vi "Set PPMS parameter.vi"(8 "error in (no error)":errorcluster, 9 "Input Value":variant, 10 "Control Name":string, 11 "VI reference in":refnum<vi>) -> (0 "error out":errorcluster, 3 "VI reference out":refnum<vi>)   [LabVIEW 2025]
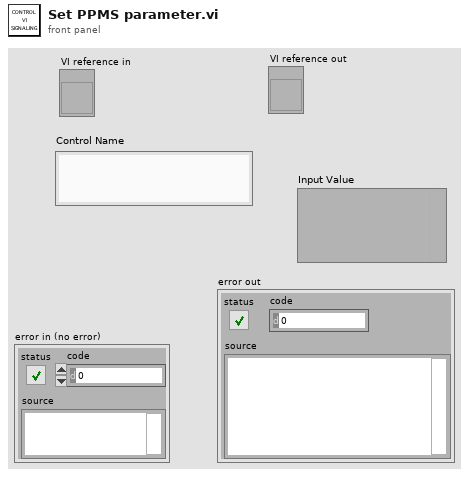
[diagram p1: front panel]
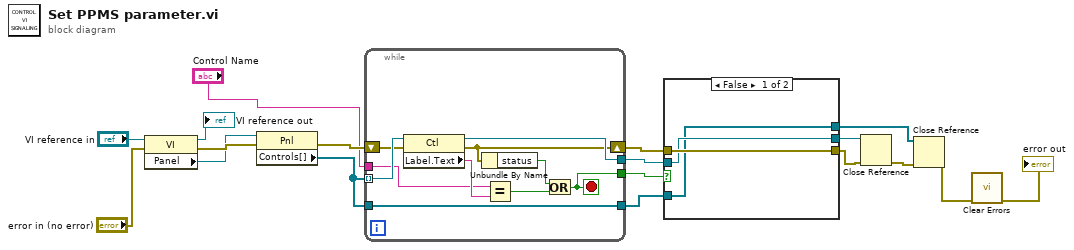
[diagram p0: block diagram]
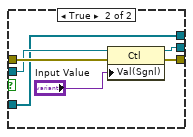
[diagram p2: hidden frame]
diagram:
  n1 = property class="VI"(reference="VI reference in", error in="error in (no error)") -> (reference out=→"VI reference out":refnum<vi>, error out=w18:errorcluster, "Panel"=w11:refnum<vi>)
  n2 = property class="Pnl"(reference=w11, error in=w18) -> (error out=w17:errorcluster, "Controls[]"=w13:refnum<vi>[])  [unwired: 1 out]
  n3 = while {
    tunnel: w13 -> [w28] mode=indexing
    tunnel: "Control Name" -> [w26]
    shift-right: [w23] -> w14
    shift-left: w17 -> [w25]
    tunnel: [w24] -> w16
    tunnel: [w20] -> w15
    tunnel: w13 -> [w19]
    tunnel: [w19] -> w12
    stop <- w20 stop-if-true
    n4 = property class="Ctl"(reference=w28, error in=w25) -> (reference out=w24:refnum<vi>, error out=w23:errorcluster, "Label.Text"=w27:string)
    n5 = Unbundle By Name(w23) -> ("status"=w22:bool)
    n6 = Equal?(x=w26, y=w27) -> (x = y?=w21:bool)
    n7 = Or(x=w22, y=w21) -> (x .or. y?=w20:bool)
  }
  n8 = case shown="False" w15 {
    tunnel: w16 -> [w30 w36]
    tunnel: w14 -> [w31 w37]
    tunnel: [w31 w34] -> w4
    tunnel: [w30 w33] -> w6
    tunnel: w12 -> [w29 w32]
    tunnel: [w29 w32] -> w5
    frame False {
    }
    frame True {
      n9 = property class="Ctl"(reference=w36, error in=w37, "Val(Sgnl)"="Input Value") -> (reference out=w33:refnum<vi>, error out=w34:errorcluster)
    }
  }
  n10 = Close Reference(reference=w6, error in (no error)=w4) -> (error out=w7:errorcluster)
  n11 = Close Reference(reference=w5, error in (no error)=w7) -> (error out=w3:errorcluster)
  n12 = call <vilib>:"Clear Errors.vi"("error in (no error)"=w3) -> ("error out"=→"error out":errorcluster)  [unwired: 5 in, 1 out]
